vi "xml_test.vi"() -> ()   [LabVIEW 2010]
uses:
  <vilib>/Utility/xml.llb/Read From XML File(string).vi
  <vilib>/Utility/xml.llb/Write to XML File(string).vi
panel:
  in  "Ring":u16(ring) items=["Read", "Write"]
  out "String":string
  out "Cluster 2":T1
  in  "Cluster":T1
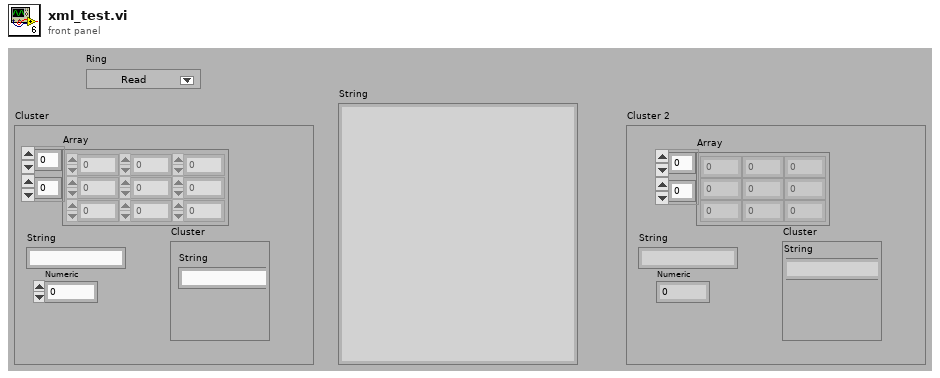
[diagram p1: front panel]
types:
  T1 = cluster{"Array":dbl[][], "String":string, "Numeric":dbl, "Cluster":cluster{"String":string}}
  T2 = cluster{"Array":dbl[][], "String":string, "Numeric":dbl, "Cluster":cluster{"String 2":string}}
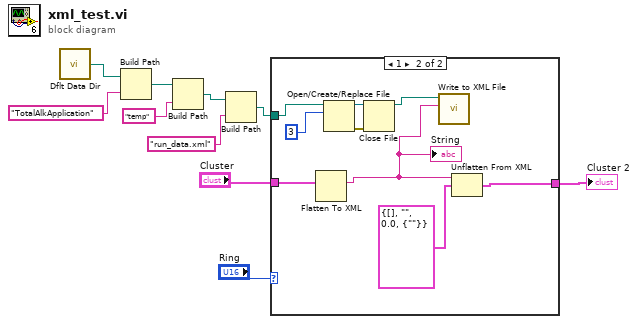
[diagram p0: block diagram]
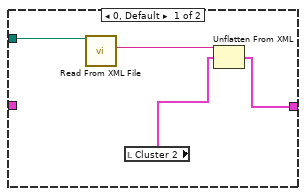
[diagram p2: hidden frame]
diagram:
  n1 = call <vilib>:"Dflt Data Dir.vi"() -> ("App:Default Data Directory"=w2:path)
  n2 = Build Path(base path=w2, name or relative path="TotalAlkApplication") -> (appended path=w6:path)
  n3 = Build Path(base path=w6, name or relative path="temp") -> (appended path=w4:path)
  n4 = Build Path(base path=w4, name or relative path="run_data.xml") -> (appended path=w1:path)
  n5 = case shown="1" "Ring" {
    tunnel: [w11 w23] -> w10
    tunnel: "Cluster" -> [_ w22]
    tunnel: w1 -> [w14 w20]
    frame 0, Default {
      n6 = call-poly <vilib>:"Read From XML File.vi"("XML File Path"=w14) -> ("XML Elements"=w12:string)  [unwired: 8 in, 2 out]
      n7 = local read "Cluster 2"() -> (w13:T1)
      n8 = Unflatten From XML(xml string=w12, type=w13) -> (value=w11:T1)  [unwired: 1 in, 1 out]
    }
    frame 1 {
      n9 = Flatten To XML(anything=w22) -> (xml string=w16:string)
      "String" <- w16
      n10 = Open/Create/Replace File(file path (use dialog)=w20, operation (0:open)=3) -> (refnum out=w18:refnum<file>, error out=w19:errorcluster)  [unwired: 4 in, 1 out]
      n11 = Close File(refnum=w18, error in=w19) -> (path=w17:path)  [unwired: 1 out]
      n12 = call-poly <vilib>:"Write to XML File.vi"("XML Input"=w16, "XML File Path"=w17) -> ()  [unwired: 7 in, 3 out]
      n13 = Unflatten From XML(xml string=w16, type=T2 {"Array"=[], "String"="", "Numeric"=0.0, "Cluster"={"String 2"=""}} ("Cluster 3")) -> (value=w23:T2)  [unwired: 1 in, 1 out]
    }
  }
  "Cluster 2" <- w10
